vi "Do.vi"(8 "error in":errorcluster, 10 "Actor in":refnum<class "Actor.lvclass">, 11 "Change Sequence State MSG":refnum<class "Change Sequence State MSG.lvclass">) -> (0 "error out":errorcluster, 2 "Actor out":refnum<class "Actor.lvclass">)   [LabVIEW 2017, in "Controller.lvlib" / "Change Sequence State MSG.lvclass"]
doc: "(<B>Filename</B>: Actor Framework.lvlib:Message.lvclass:Do.vi)\n\nDefines what a message does when it is received by an actor. Generally, a message instructs an actor to invoke one of its methods. By default, this method does nothing. A child class must override it to define behavior. Create a child class by using the Actor Framework Message Maker dialog box."
uses:
  Change Sequence State MSG.lvclass
  <vilib>/ActorFramework/Actor/Actor.lvclass
  Change Sequence State MSG.lvclass/Change Sequence State MSG.ctl
  gController.lvclass
  C:/Program Files (x86)/National Instruments/LabVIEW 2017/vi.lib/MSR Consulting, LLC/General Reuse/SuperActor/SuperActor.lvclass
  C:/Program Files (x86)/National Instruments/LabVIEW 2017/vi.lib/ActorFramework/Actor/Actor.lvclass
  <vilib>/MSR Consulting, LLC/General Reuse/SuperActor/SuperActor.lvclass/SuperActor.ctl
  gController.lvclass/gController.ctl
  <vilib>/MSR Consulting, LLC/General Reuse/SuperActor/Read Log Session.vi
  Read seq_state.vi
  <vilib>/MSR Consulting, LLC/General Reuse/SuperActor/Read CVT Session.vi
  <vilib>/MSR Consulting, LLC/General Reuse/Session APIs/_Session Fwk/Session - Root.lvclass
  <vilib>/MSR Consulting, LLC/General Reuse/Session APIs/Session Log/System Log.lvclass
  <vilib>/MSR Consulting, LLC/General Reuse/Session APIs/CVT/CVT.lvclass
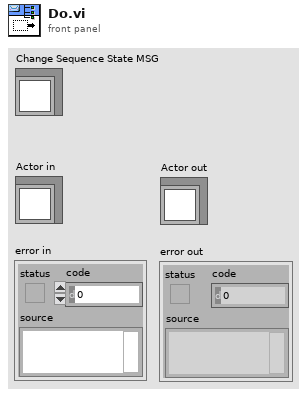
[diagram p1: front panel]
types:
  T1 = typedef "Controller.lvlib/sequenceState.ctl" = enum16{"Run", "Pause", "Reset", "Reload", "Stop"}
  T2 = typedef "Session - Root.lvclass/Session Handle.ctl" = refnum<data-value>
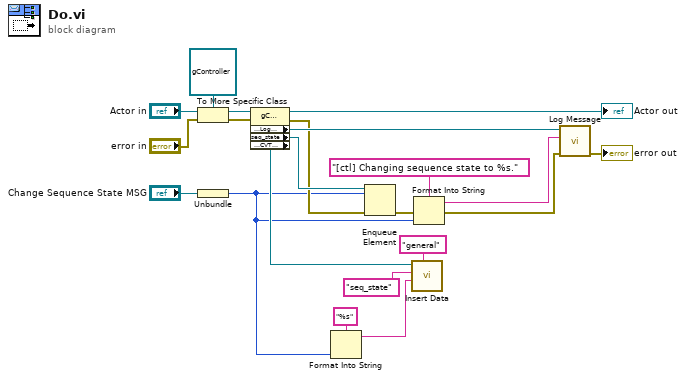
[diagram p0: block diagram]
diagram:
  n1 = To More Specific Class(target class=refnum<class "gController.lvclass"> refnum ("Controller.lvlib:gController"), reference="Actor in", error in="error in") -> (specific class reference=w19:refnum<class "gController.lvclass">, error out=w13:errorcluster)
  n2 = Unbundle("Change Sequence State MSG") -> (w5:T1)
  n3 = property class="gController"(reference=w19, error in=w13) -> (reference out=→"Actor out":refnum<class "gController.lvclass">, error out=w12:errorcluster, "Accessors:Log Session"=w14:T2, "seq_state"=w15:refnum<queue>, "Accessors:CVT Session"=w6:T2)
  n4 = Format Into String(format string="%s", w5) -> (resulting string=w3:string)  [unwired: 2 in, 1 out]
  n5 = Enqueue Element(queue=w15, element=w5, error in (no error)=w12) -> (error out=w11:errorcluster)  [unwired: 1 in, 2 out]
  n6 = call <vilib>:"Insert Data.vi"("Group"="general", "Data"=w3, "tag"="seq_state", "CVT Session In"=w6) -> ()  [unwired: 6 in, 2 out]
  n7 = Format Into String(format string="[ctl] Changing sequence state to %s." ("initial string"), error in=w11, w5) -> (resulting string=w7:string, error out=w8:errorcluster)  [unwired: 1 in]
  n8 = call <vilib>:"Log Message.vi"("error in"=w8, "MSG In"=w7, "session in"=w14) -> ("error out"=→"error out":errorcluster)  [unwired: 7 in, 1 out]
